vi "Write Binary Data.vi"(8 "error in (no error)":errorcluster, 10 "Send Binary Data":u8[](array[numeric]), 11 "WebSocket Client CR in":refnum<class "WebSocket Client CR.lvclass">) -> (0 "error out":errorcluster)   [LabVIEW 2021, in "WebSockets.lvlib" / "WebSocket Client CR.lvclass"]
uses:
  WebSocket Client CR.lvclass
  WebSocket Client CR.lvclass/WebSocket Client CR.ctl
  Modbus_v121c/Data Model/Device Data Model.lvclass
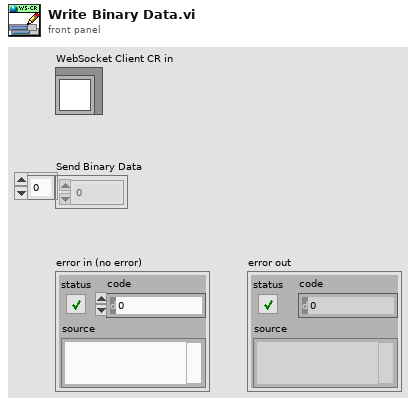
[diagram p1: front panel]
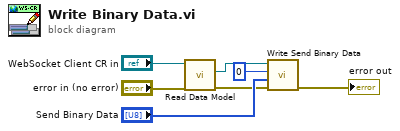
[diagram p0: block diagram]
diagram:
  n1 = call "Read Data Model.vi"("error in (no error)"="error in (no error)", "Master CR in"="WebSocket Client CR in") -> ("error out"=w4:errorcluster, "Data Model"=w5:refnum<class "Device Data Model.lvclass">)  [unwired: 7 in, 1 out]
  n2 = call-dynamic "Write Send Binary Data.vi"("error in (no error)"=w4, "values"="Send Binary Data", "starting address"=u16 0, "standard data model in"=w5) -> ("error out"=→"error out":errorcluster)  [unwired: 6 in, 1 out]
